vi "CheckUserPassword_SN.vi"(3 "error in (no error)":errorcluster, 4 "Password":string, 5 "User name":string, 6 "Arr_LoginDetails":string[][](array[string])) -> (0 "error out":errorcluster, 1 "PermissionLevel":string, 2 "Bool_LoginTrue":bool)   [LabVIEW 2012]
panel:
  # "Function used to check user name and Password exists in configured file returen true if the text matches"
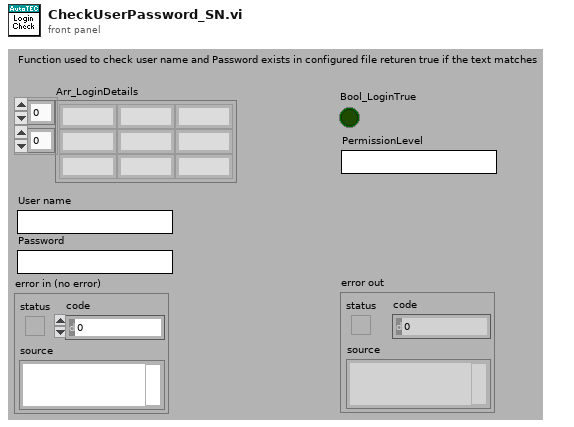
[diagram p1: front panel]
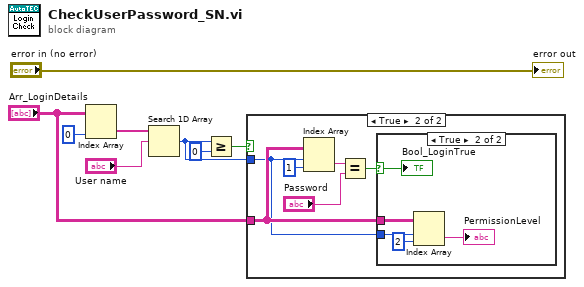
[diagram p0: block diagram]
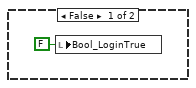
[diagram p2: hidden frame]
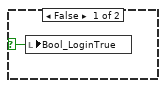
[diagram p3: hidden frame]
diagram:
  n1 = Index Array(array="Arr_LoginDetails", index (col)=0 ("disabled index (col)")) -> (element=w7:string[])  [unwired: 1 in]
  n2 = Search 1D Array(1D array=w7, element="User name") -> (index of element=w4:i32)  [unwired: 1 in]
  n3 = Greater Or Equal?(x=w4, y=0) -> (x >= y?=w5:bool)
  n4 = case shown="True" w5 {
    tunnel: "Arr_LoginDetails" -> [_ w12]
    tunnel: w4 -> [_ w11]
    frame False {
      n5 = local write "Bool_LoginTrue"(FALSE ("Bool_LoginTrue")) -> ()
    }
    frame True {
      n6 = Index Array(array=w12, index (row)=w11, index (col)=1 ("disabled index (col)")) -> (element=w14:string)
      n7 = Equal?(x=w14, y="Password") -> (x = y?=w13:bool)
      n8 = case shown="True" w13 {
        selector: w13 -> [w16 w17]
        tunnel: w12 -> [_ w21]
        tunnel: w11 -> [_ w20]
        frame False {
          n9 = local write "Bool_LoginTrue"(w16) -> ()
        }
        frame True {
          n10 = Index Array(array=w21, index (row)=w20, index (col)=2 ("disabled index (col)")) -> (element=→"PermissionLevel":string)
          "Bool_LoginTrue" <- w17
        }
      }
    }
  }
  "error out" <- "error in (no error)"
